vi "Start Memory Sweep.vi"(8 "error in (no error)":errorcluster, 9 "Number of Points (5)":u32=5, 10 "Starting Memory Location (1)":u32=1, 11 "VISA resource name":refnum<visa-resource-name>) -> (0 "error out":errorcluster, 3 "VISA resource name out":refnum<visa-resource-name>)   [LabVIEW 2017, in "Keithley 24XX.lvlib"]
doc: "Begins a memory sweep operation for running configurations in multiple memory blocks.\n\n<B>Note:</B> This VI calls Initiate, so the Initiate VI should not be used to start a memory sweep."
uses:
  Keithley 24XX.lvlib
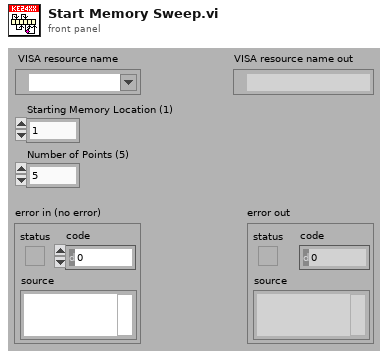
[diagram p1: front panel]
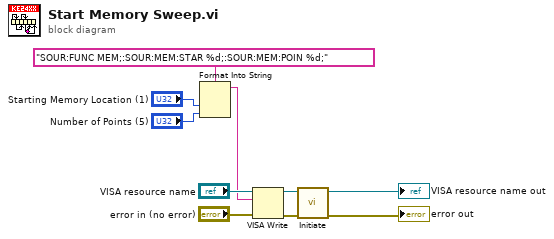
[diagram p0: block diagram]
diagram:
  n1 = Format Into String(format string="SOUR:FUNC MEM;:SOUR:MEM:STAR %d;:SOUR:MEM:POIN %d;", "Starting Memory Location (1)", "Number of Points (5)") -> (resulting string=w5:string)  [unwired: 2 in, 1 out]
  n2 = VISA Write(VISA resource name="VISA resource name", write buffer=w5, error in (no error)="error in (no error)") -> (VISA resource name out=w4:refnum<visa-resource-name>, error out=w3:errorcluster)  [unwired: 1 out]
  n3 = call "Initiate.vi"("error in (no error)"=w3, "VISA resource name"=w4) -> ("error out"=→"error out":errorcluster, "VISA resource name out"=→"VISA resource name out":refnum<visa-resource-name>)  [unwired: 8 in]
